vi "rx streamer make.vi"(8 "error in (no error)":errorcluster, 11 "h 2":u64) -> (0 "error out":errorcluster, 2 "function return":u32(ring), 3 "h 3":u64)   [LabVIEW 2023, in "uhd.lvlib"]
doc: "UHD_API uhd_error uhd_rx_streamer_make(uhd_rx_streamer_handle* h);"
uses:
  <userlib>/uhd/uhd.lvlib
  <userlib>/uhd/uhd.dll
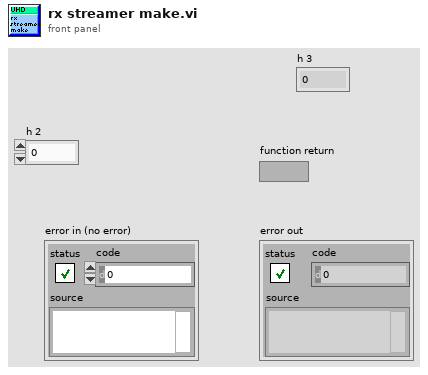
[diagram p1: front panel]
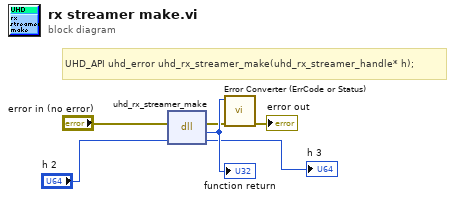
[diagram p0: block diagram]
diagram:
  # "UHD_API uhd_error uhd_rx_streamer_make(uhd_rx_streamer_handle* h);"
  n1 = dll-call lib="C:/Program Files/National Instruments/LabVIEW 2023/user.lib/uhd/uhd.*" fn="uhd_rx_streamer_make"(error in="error in (no error)", "h"="h 2") -> (error out=w4:errorcluster, w6:u32, "h"=→"h 3":u64)  [unwired: 2 in, 1 out]
  "function return" <- w6
  n2 = call <userlib>:"Error Converter (ErrCode or Status).vi"("error in (no error)"=w4, "error code"=w6) -> ("error out"=→"error out":errorcluster)  [unwired: 9 in]
